vi "TCP Client_21.vi"() -> ()   [LabVIEW 2021]
panel:
  out "data string":string
  out "Data string length: bytes written":i32
  in  "data wrote":string
  out "value 2":cluster{i32}
  out "value":cluster{i32}
  out "Received":string
  in  "remote port or service name":u16
  in  "address":string
  in  "Stop":bool
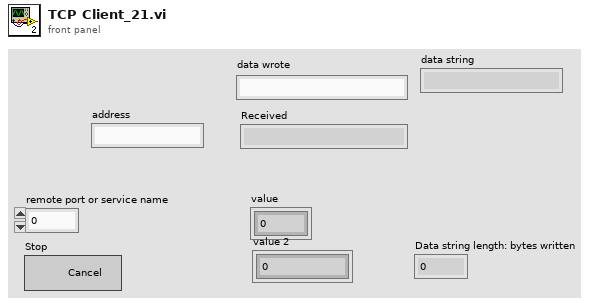
[diagram p1: front panel]
types:
  T1 = enum16{"big-endian, network order", "native, host order", "little-endian"}
  T2 = enum16{"Standard", "Buffered", "CRLF", "Immediate"}
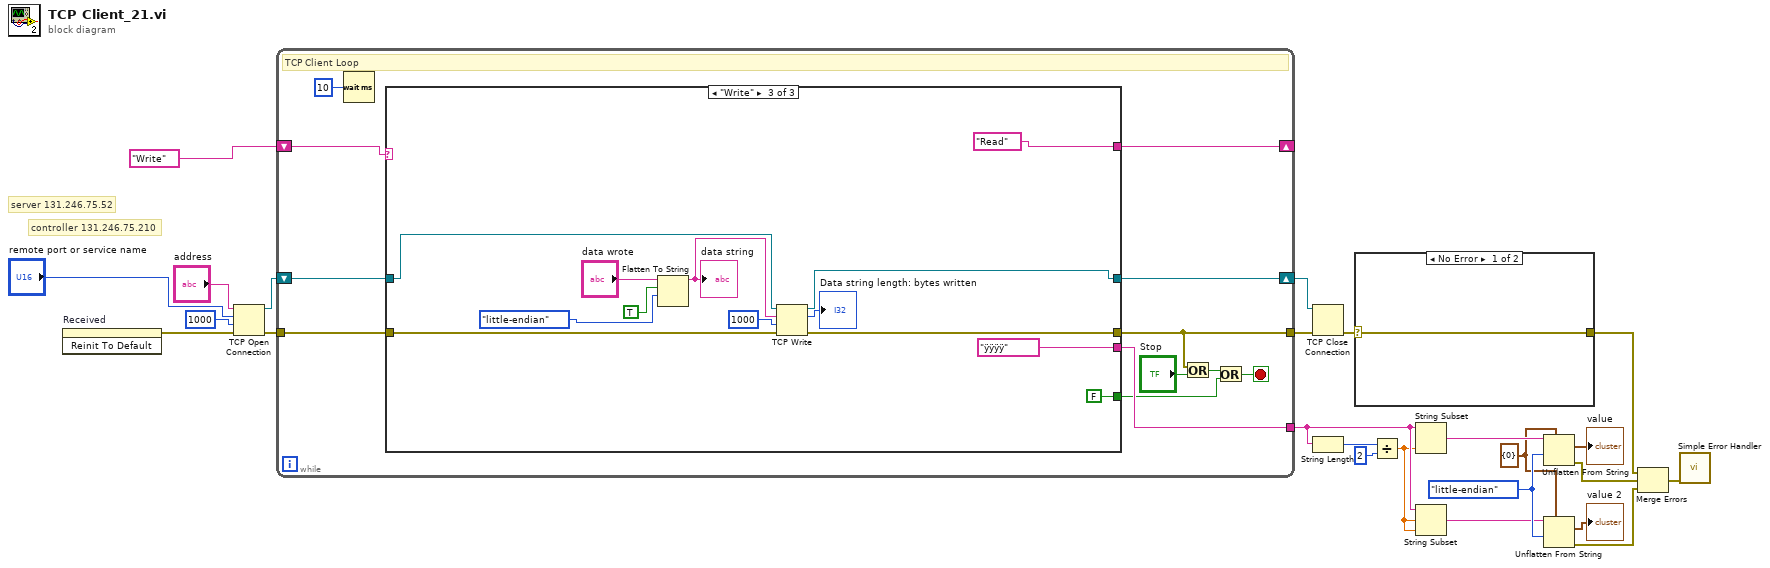
[diagram p0: block diagram]
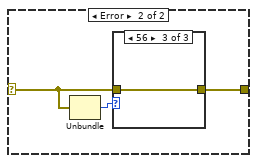
[diagram p2: hidden frame]
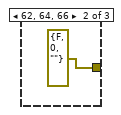
[diagram p4: hidden frame]
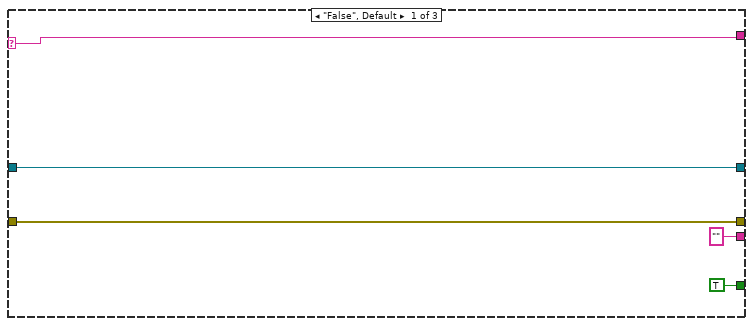
[diagram p5: hidden frame]
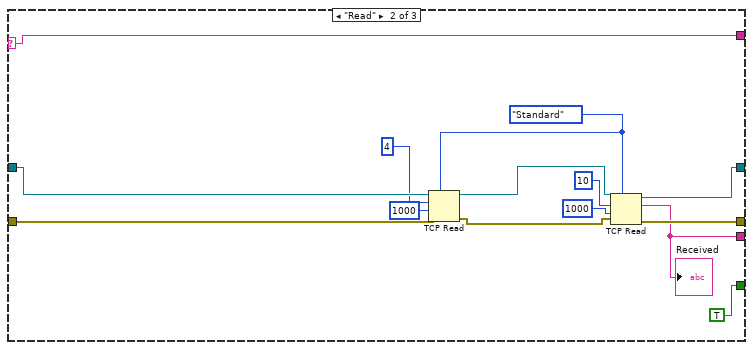
[diagram p6: hidden frame]
diagram:
  w8 = cluster{i32} {0} ("type")
  w11 = T1."little-endian" ("byte order (0:big-endian, network order)")
  # "controller 131.246.75.210"
  # "server 131.246.75.52"
  n1 = invoke on="Received" class="Str" method="Reinit To Default"() -> (error out=w18:errorcluster)  [unwired: 3 in, 2 out]
  n2 = TCP Open Connection(address="address", remote port or service name="remote port or service name", timeout ms (60000)=1000, error in (no error)=w18) -> (connection ID=w17:refnum<k5>, error out=w24:errorcluster)  [unwired: 1 in]
  n3 = while {
    tunnel: w24 -> [w32]
    tunnel: [w33] -> w22
    shift-right: [w34] -> w20
    shift-left: w17 -> [w31]
    tunnel: [w30] -> w16
    shift-right: [w25] -> _
    shift-left: "Write" ("Combo Box") -> [w26]
    stop <- w28 stop-if-true
    # "TCP Client Loop"
    n4 = Wait (ms)(milliseconds to wait=u32 10) -> ()  [unwired: 1 out]
    n5 = case shown="\"Write\"" w26 {
      selector: w26 -> [w37 w49 _]
      tunnel: [w41 w55 w58] -> w34
      tunnel: [w40 w54 w59] -> w33
      tunnel: w32 -> [w40 w48 w68]
      tunnel: w31 -> [w41 w46 w67]
      tunnel: ["" ("data out") w51 "ÿÿÿÿ" ("data out")] -> w30
      tunnel: [TRUE TRUE FALSE] -> w29
      tunnel: [w37 w49 "Read" ("Combo Box")] -> w25
      frame "False", Default {
      }
      frame "Read" {
        w43 = T2."Standard" ("mode (standard)")
        n6 = TCP Read(connection ID=w46, bytes to read=4, error in (no error)=w48, 7:w43, 9:1000 ("timeout ms (25000)")) -> (connection ID out=w45:refnum<k5>, error out=w47:errorcluster)  [unwired: 1 out]
        n7 = TCP Read(connection ID=w45, bytes to read=10, error in (no error)=w47, 7:w43, 9:1000 ("timeout ms (25000)")) -> (connection ID out=w55:refnum<k5>, data out=w51:string, error out=w54:errorcluster)
        "Received" <- w51
      }
      frame "Write" {
        n8 = Flatten To String(anything="data wrote", prepend array or string size? (T)=TRUE, byte order (0:big-endian, network order)=T1."little-endian") -> (data string=w57:string)  [unwired: 1 in, 2 out]
        "data string" <- w57
        n9 = TCP Write(connection ID=w67, data in=w57, error in (no error)=w68, 9:1000 ("timeout ms (25000)")) -> (connection ID out=w58:refnum<k5>, bytes written=→"Data string length: bytes written":i32, error out=w59:errorcluster)
      }
    }
    n10 = Or(x=w33, y="Stop") -> (x .or. y?=w27:bool)
    n11 = Or(x=w27, y=w29) -> (x .or. y?=w28:bool)
  }
  n12 = TCP Close Connection(connection ID=w20, error in (no error)=w22) -> (error out=w21:errorcluster)  [unwired: 1 in, 1 out]
  n13 = String Length(string=w16) -> (length=w15:i32)
  n14 = case shown="No Error" w21 {
    selector: w21 -> [w69 w71]
    tunnel: [w69 w70] -> w4
    frame No Error {
    }
    frame Error {
      n15 = Unbundle(w71) -> ("code"=w72:i32)  [unwired: 2 out]
      n16 = case shown="56" w72 {
        tunnel: [w73 errorcluster {"status"=FALSE, "code"=0, "source"=""} ("error IO") w75] -> w70
        tunnel: w71 -> [w73 _ w75]
        frame 0, Default {
        }
        frame 62, 64, 66 {
        }
        frame 56 {
        }
      }
    }
  }
  n17 = Divide(x=w15, y=2) -> (x/y=w13:dbl)
  n18 = String Subset(string=w16, length (rest)=w13) -> (substring=w12:string)  [unwired: 1 in]
  n19 = String Subset(string=w16, offset (0)=w13, length (rest)=w13) -> (substring=w7:string)
  n20 = Unflatten From String(type=w8, binary string=w12, byte order (0:big-endian, network order)=w11) -> (value=→"value":cluster{i32}, error out=w6:errorcluster)  [unwired: 2 in, 1 out]
  n21 = Unflatten From String(type=w8, binary string=w7, byte order (0:big-endian, network order)=w11) -> (value=→"value 2":cluster{i32}, error out=w5:errorcluster)  [unwired: 2 in, 1 out]
  n22 = Merge Errors(w4, w6, w5) -> (w3:errorcluster)
  n23 = call <vilib>:"Simple Error Handler.vi"("error in (no error)"=w3) -> ()  [unwired: 4 in, 5 out]
